vi "_FPGA Set Oscillator.vi"(4 "Param 3":u32, 5 "error in":errorcluster, 6 "Param 2":u32, 7 "Param 1":u32) -> (0 "error out":errorcluster)   [LabVIEW 2015]
uses:
  Type/_FPGA Indicator.ctl
  _RT Global.vi
  <vilib>/Utility/error.llb/Error Cluster From Error Code.vi
  <vilib>/rvi/errors/niLvFpgaAdjustHostInterfaceError.vi
  <vilib>/rvi/interface/nirviReadWriteControl/nirviReadWriteControl.xnode
  Type/FPGA Typedef.ctl
  FPGA Bitfiles/FPGA9607.lvbitx
  NiFpgaLv.dll
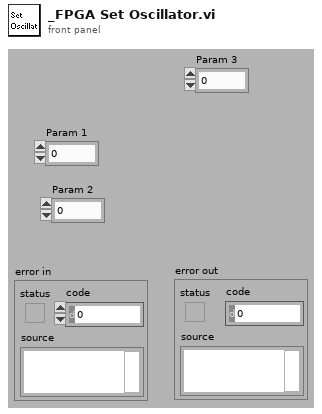
[diagram p1: front panel]
types:
  T1 = typedef "Semaphore RefNum" = refnum<k1>
  T2 = typedef "_FPGA Indicator.ctl" = enum16{"Done", "Ready", "Count Available", "SendSerial", "LED State"}
  T3 = typedef "FPGA Typedef.ctl" = refnum<k20>
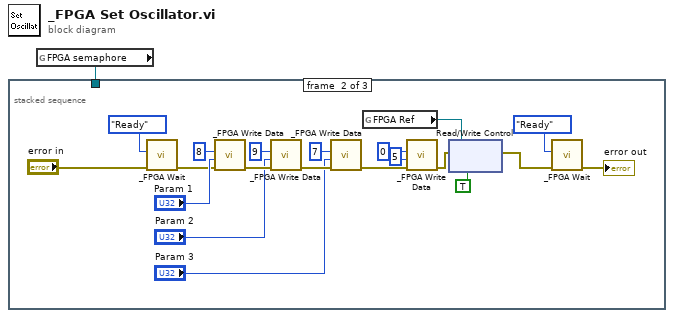
[diagram p0: block diagram]
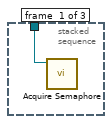
[diagram p2: hidden frame]
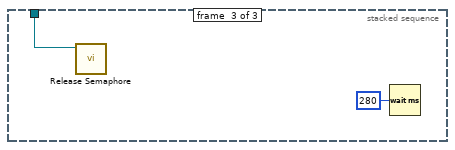
[diagram p3: hidden frame]
diagram:
  n1 = global read "_RT Global.vi" "FPGA semaphore"() -> (w1:T1)
  n2 = stacked-sequence {
    tunnel: w1 -> [w2 _ w24]
    frame #0 {
      n3 = call <vilib>:"Acquire Semaphore.vi"("semaphore"=w2) -> ()  [unwired: 2 in, 5 out]
    }
    frame #1 {
      n4 = call "_FPGA Wait.vi"("error in"="error in", "Indicator"=_FPGA_Indicator."Ready") -> ("error out"=w5:errorcluster)  [unwired: 3 in, 2 out]
      n5 = call "_FPGA Write Data.vi"("error in"=w5, "Data"="Param 1", "Address"=u16 8) -> ("error out"=w22:errorcluster)  [unwired: 3 in, 2 out]
      n6 = call "_FPGA Write Data.vi"("error in"=w22, "Data"="Param 2", "Address"=u16 9) -> ("error out"=w12:errorcluster)  [unwired: 3 in, 2 out]
      n7 = call "_FPGA Write Data.vi"("error in"=w12, "Data"="Param 3", "Address"=u16 7) -> ("error out"=w10:errorcluster)  [unwired: 3 in, 2 out]
      n8 = global read "_RT Global.vi" "FPGA Ref"() -> (w3:T3)
      n9 = call "_FPGA Write Data.vi"("error in"=w10, "Data"=u32 5 ("Address"), "Address"=u16 0) -> ("error out"=w17:errorcluster)  [unwired: 3 in, 2 out]
      n10 = xnode "Read/Write Control"("FPGA VI Reference In"=w3, "error in"=w17, "Start"=TRUE) -> ("error out"=w8:errorcluster)  [unwired: 1 out]
      n11 = call "_FPGA Wait.vi"("error in"=w8, "Indicator"=_FPGA_Indicator."Ready") -> ("error out"=→"error out":errorcluster)  [unwired: 3 in, 2 out]
    }
    frame #2 {
      n12 = call <vilib>:"Release Semaphore.vi"("semaphore"=w24) -> ()  [unwired: 1 in, 6 out]
      n13 = Wait (ms)(milliseconds to wait=u32 280) -> ()  [unwired: 1 out]
    }
  }
